vi "ButtonSinglePress.vi"(11 "Button In":bool) -> (3 "Button out":bool)   [LabVIEW 2015]
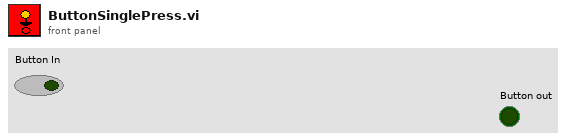
[diagram p1: front panel]
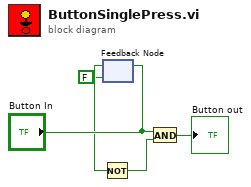
[diagram p0: block diagram]
diagram:
  n1 = feedback-in #1("Button In") -> ()
  n2 = feedback #1(FALSE ("Button In")) -> (w2:bool)
  n3 = Not(x=w2) -> (.not. x?=w5:bool)
  n4 = And(x="Button In", y=w5) -> (x .and. y?=→"Button out":bool)
